vi "PulseStretch.vi"(6 "state in":T1={"input"=TRUE, "output"=TRUE, "pulse count"=0}, 7 "Reset":bool, 9 "Pulse Width":i32, 11 "Input":bool) -> (3 "Output":bool, 4 "state out":T1={"input"=TRUE, "output"=TRUE, "pulse count"=0})   [LabVIEW 2017, in "cRIOWfmLib.lvlib"]
uses:
  <vilib>/addons/InsightCM/Devices/Shared/Cms/cRIOWfmAcq/cRIOWfmLib.lvlib
  <vilib>/addons/InsightCM/Devices/Shared/Cms/cRIOWfmAcq/subVIs/stretchState.ctl
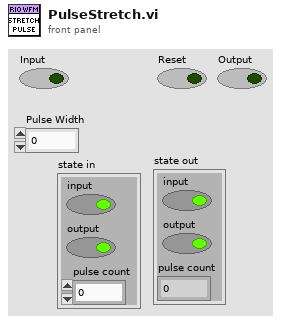
[diagram p1: front panel]
types:
  T1 = typedef "cRIOWfmLib.lvlib/stretchState.ctl" = cluster{"input":bool, "output":bool, "pulse count":i32}
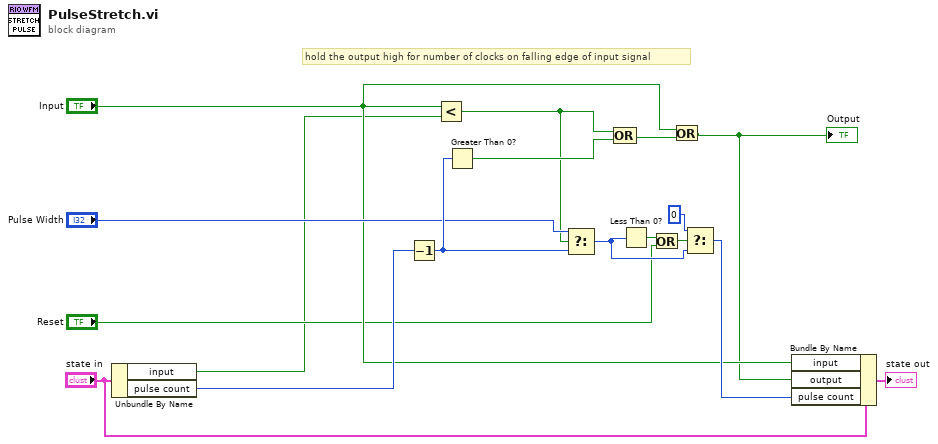
[diagram p0: block diagram]
diagram:
  # "hold the output high for number of clocks on falling edge of input signal"
  n1 = Unbundle By Name("state in") -> ("input"=w1:bool, "pulse count"=w7:i32)
  n2 = Decrement(x=w7) -> (x-1=w17:i32)
  n3 = Less?(x="Input", y=w1) -> (x < y?=w3:bool)
  n4 = Greater Than 0?(x=w17) -> (x > 0?=w11:bool)
  n5 = Select(t="Pulse Width", s=w3, f=w17) -> (s? t:f=w16:i32)
  n6 = Compound Arithmetic op=OR(w3, w11) -> (w6:bool)
  n7 = Less Than 0?(x=w16) -> (x < 0?=w13:bool)
  n8 = Or(x=w13, y="Reset") -> (x .or. y?=w14:bool)
  n9 = Or(x="Input", y=w6) -> (x .or. y?=w4:bool)
  "Output" <- w4
  n10 = Select(t=0, s=w14, f=w16) -> (s? t:f=w9:i32)
  n11 = Bundle By Name(cluster="state in", "input"="Input", "output"=w4, "pulse count"=w9) -> (→"state out":T1)
